vi "List Mode - Seq - Configure Current Low Limitation.vi"(8 "error in (no error)":errorcluster, 10 "A-LO":dbl min=0.0 max=30.0, 11 "VISA resource name":refnum<visa-resource-name>) -> (0 "error out":errorcluster, 3 "VISA resource name out":refnum<visa-resource-name>)   [LabVIEW 2014, in "Associated Power Technologies 8500 Series.lvlib"]
doc: "Configure the current low limitation in sequence.\n\n<B>Note: Couple = AC mode max current</B>\nAPT-8505 Low: 5A@100V High: 2.5A 200V\nAPT-8512 Low: 12.5A@100V High: 6.25A@200V\nAPT-8520 Low: 20A@100V High: 10A@200V\nAPT-8540 Low: 40A@100V High: 20A@200V\n\n<B>Note: Couple = DC mode max current</B>\nAPT-8505 Low: 3A High: 1.5A\nAPT-8512 Low: 7.5A High: 3.75A\nAPT-8520 Low: 12A High: 6A\nAPT-8540 Low: 24A High: 12A\n\nDefault value: 0 (OFF)"
uses:
  <instrlib>/Associated Power Technologies 8500 Series/Associated Power Technologies 8500 Series.lvlib
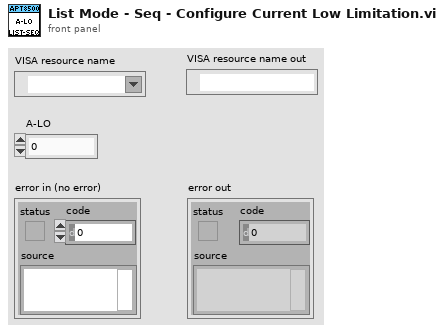
[diagram p1: front panel]
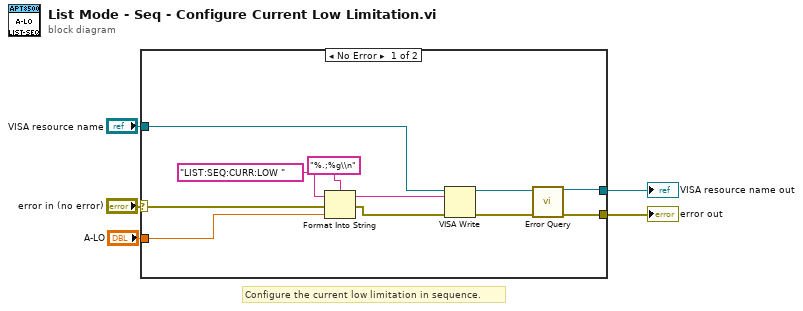
[diagram p0: block diagram]
diagram:
  # "Configure the current low limitation in sequence."
  n1 = case shown="No Error" "error in (no error)" {
    selector: "error in (no error)" -> [w15 w17]
    tunnel: "A-LO" -> [w16 _]
    tunnel: "VISA resource name" -> [w11 w18]
    tunnel: [w8 w18] -> w2
    tunnel: [w6 w17] -> w1
    frame No Error {
      n2 = Format Into String(format string="%.;%g\\n", initial string="LIST:SEQ:CURR:LOW " ("command"), error in=w15, w16) -> (resulting string=w10:string, error out=w14:errorcluster)
      n3 = VISA Write(VISA resource name=w11, write buffer=w10, error in (no error)=w14) -> (VISA resource name out=w9:refnum<visa-resource-name>, error out=w7:errorcluster)  [unwired: 1 out]
      n4 = call <instrlib>:"Error Query.vi"("VISA resource name"=w9, "error in (no error)"=w7) -> ("VISA resource name out"=w8:refnum<visa-resource-name>, "error out"=w6:errorcluster)  [unwired: 10 in, 2 out]
    }
    frame Error {
    }
  }
  "VISA resource name out" <- w2
  "error out" <- w1
